vi "PrepareChannels_v2.vi"(0 "AO Physical channels":tag="pciDAQ/ao0", 1 "Sampling Rate (Hz)":dbl=100000.0, 2 "Onboard counter":tag="pciDAQ/ctr0", 5 "DO Physical channels":tag="pciDAQ/port0/line1:2", 7 "OEP sample clock in":tag="/pciDAQ/PFI0", 9 "Num Pulses":u32=1 min=1, 11 "Pulse Width (ms)":dbl=0.09, 14 "Pulse Type":enum16{"Monophasic", "Biphasic"}(ring)=enum."Biphasic") -> (3 "Waveform Graph":waveform(dbl)(graph), 4 "AO task out":refnum<k21>, 6 "AO error out":errorcluster, 10 "ctr task out":refnum<k21>, 12 "DO error out":errorcluster, 13 "DO task out":refnum<k21>, 15 "ctr error out":errorcluster)   [LabVIEW 2017]
uses:
  <vilib>/DAQmx/write.llb/DAQmx Write (Analog Wfm 1Chan NSamp).vi
  <vilib>/DAQmx/create/channels.llb/DAQmx Create Channel (DO-Digital Output).vi
  <vilib>/DAQmx/miscellaneous.llb/DAQmx Fill In Error Info.vi
  <vilib>/DAQmx/configure/timing.llb/DAQmx Timing (Use Waveform).vi
  <vilib>/DAQmx/create/channels.llb/DAQmx Create Channel (AO-Voltage-Basic).vi
  <vilib>/DAQmx/create/channels.llb/DAQmx Create Channel (CI-Count Edges).vi
  <resource>/objmgr/daqmx.rc
panel:
  in  "Amplitude (Volts)":dbl=1.0
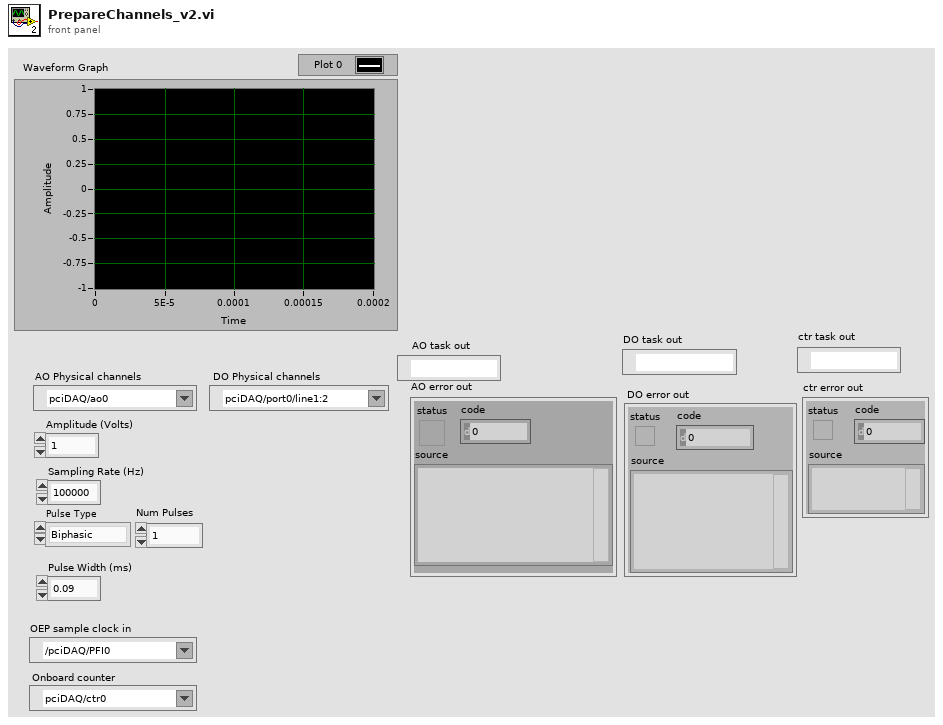
[diagram p1: front panel]
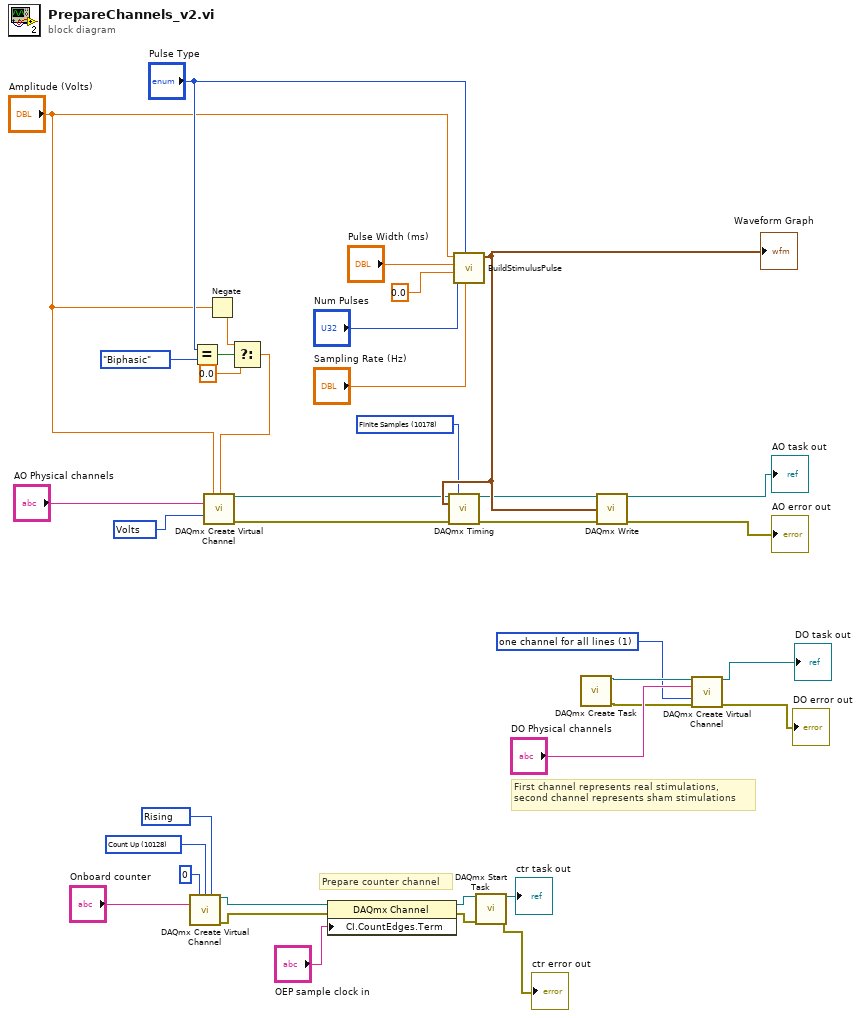
[diagram p0: block diagram]
diagram:
  w8 = 10280 items=["Rising"=10280, "Falling"=10171] ("edge")
  w9 = 10128 items=["Count Up"=10128, "Count Down"=10124, "Externally Controlled"=10326] ("count direction")
  w24 = 10178 items=["Finite Samples"=10178, "Continuous Samples"=10123, "Hardware Timed Single Point"=12522] ("sample mode")
  w29 = 10348 items=["Volts"=10348, "From Custom Scale"=10065] ("units")
  w33 = 1 items=["one channel for each line", "one channel for all lines"] ("line grouping")
  # "Prepare counter channel"
  # "First channel represents real stimulations,\nsecond channel represents sham stimulations"
  n1 = call-poly <vilib>:"DAQmx Create Virtual Channel.vi"("initial count"=u32 0, "count direction"=w9, "edge"=w8, "counter"="Onboard counter") -> ("task out"=w11:refnum<k21>, "error out"=w10:errorcluster)  [unwired: 10 in]
  n2 = Equal?(x="Pulse Type", y=enum16{"Monophasic", "Biphasic"}."Biphasic") -> (x = y?=w19:bool)
  n3 = Negate(x="Amplitude (Volts)") -> (-x=w17:dbl)
  n4 = Select(t=w17, s=w19, f=0.0) -> (s? t:f=w15:dbl)
  n5 = call-poly <vilib>:"DAQmx Create Virtual Channel.vi"("maximum value"="Amplitude (Volts)", "minimum value"=w15, "physical channels"="AO Physical channels", "units"=w29) -> ("task out"=w23:refnum<k21>, "error out"=w22:errorcluster)  [unwired: 10 in]
  n6 = property class="DAQmx Channel"(reference=w11, error in=w10, "CI.CountEdges.Term"="OEP sample clock in") -> (reference out=w7:refnum<k21>, error out=w6:errorcluster)
  n7 = call "BuildStimulusPulse.vi"("Sampling Rate (Hz)"="Sampling Rate (Hz)", "Pulse Type"="Pulse Type", "Num Pulses"="Num Pulses", "Inter-Pulse Interval (ms)"=0.0, "Pulse Width (ms)"="Pulse Width (ms)", "Amplitude (Volts)"="Amplitude (Volts)") -> ("Waveform Out"=w30:waveform(dbl))  [unwired: 3 in, 2 out]
  "Waveform Graph" <- w30
  n8 = call-poly <vilib>:"DAQmx Timing.vi"("task/channels in"=w23, "sample mode"=w24, "waveform"=w30, "error in"=w22) -> ("task out"=w14:refnum<k21>, "error out"=w13:errorcluster)  [unwired: 10 in]
  n9 = call <vilib>:"DAQmx Start Task.vi"("task/channels in"=w7, "error in"=w6) -> ("task out"=→"ctr task out":refnum<k21>, "error out"=→"ctr error out":errorcluster)  [unwired: 12 in]
  n10 = call <vilib>:"DAQmx Create Task.vi"() -> ("task out"=w37:refnum<k21>, "error out"=w36:errorcluster)  [unwired: 14 in]
  n11 = call-poly <vilib>:"DAQmx Write.vi"("task/channels in"=w14, "data"=w30, "error in"=w13) -> ("task out"=→"AO task out":refnum<k21>, "error out"=→"AO error out":errorcluster)  [unwired: 10 in, 1 out]
  n12 = call-poly <vilib>:"DAQmx Create Virtual Channel.vi"("task in"=w37, "lines"="DO Physical channels", "line grouping"=w33, "error in"=w36) -> ("task out"=→"DO task out":refnum<k21>, "error out"=→"DO error out":errorcluster)  [unwired: 10 in]
